vi "sort sample information.vi"(8 "error in (no error)":errorcluster, 11 "Group run list write":string[][](array[string])) -> (0 "array out":string[](array[string]), 2 "spreadsheet string":string, 4 "error out":errorcluster)   [LabVIEW 2016]
doc: "Gets all values for current sample running to display or put into database"
panel:
  out "current index":i32
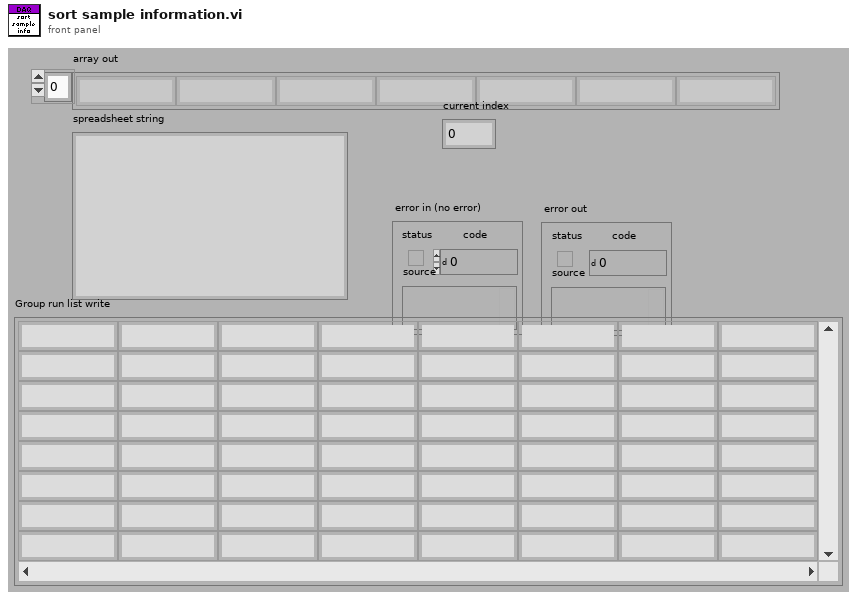
[diagram p1: front panel]
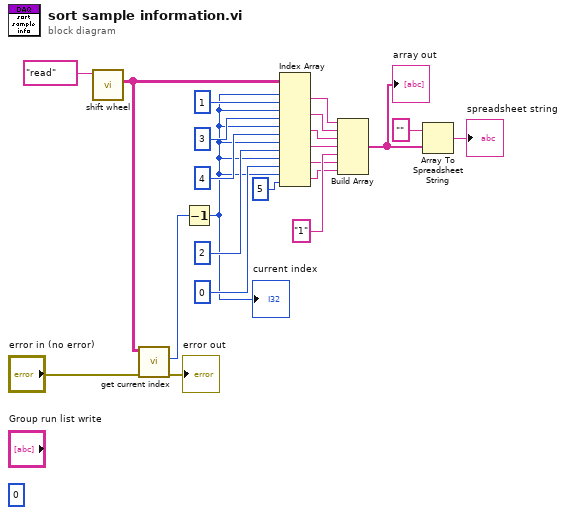
[diagram p0: block diagram]
diagram:
  (unwired) 0 ("index (row)")
  n1 = call "shift wheel.vi"("read write"="read") -> ("Group run list"=w5:string[][])  [unwired: 8 in, 2 out]
  n2 = call "get current index.vi"("error in (no error)"="error in (no error)", "Group run list in"=w5) -> ("error out"=→"error out":errorcluster, "current index"=w2:i32)  [unwired: 7 in, 1 out]
  n3 = Decrement(x=w2) -> (x-1=w1:i32)
  "current index" <- w1
  n4 = Index Array(array=w5, index (row) #1=w1, index (col) #1=1 ("disabled index (col)"), index (row) #2=w1, index (col) #2=3 ("disabled index (col)"), index (row) #3=w1, index (col) #3=4 ("disabled index (col)"), index (row) #4=w1, index (col) #4=2 ("disabled index (col)"), index (row) #5=w1, index (col) #5=0 ("disabled index (col)"), index (row) #6=w1, index (col) #6=5 ("disabled index (col)")) -> (element #1=w17:string, element #2=w16:string, element #3=w15:string, element #4=w14:string, element #5=w12:string, element #6=w11:string)
  n5 = Build Array(w17, w16, w15, w14, "1" ("element"), w12, w11) -> (w8:string[])
  "array out" <- w8
  n6 = Array To Spreadsheet String(array=w8, 3:"" ("format string")) -> (spreadsheet string=→"spreadsheet string":string)  [unwired: 1 in]
